vi "SVXMPL_Convert WDT to WAV.vi"(7 "Input range":sgl format="%.2f", 8 "error in (no error)":errorcluster, 10 "sound format":T1={"sound quality"=enum."mono", "rate"=enum."44100", "bits per sample"=enum."16 bit"}, 11 "Waveform":waveform(dbl)={"t0"=timestamp(0 s since 1904-01-01), "dt"=0.0, "Y"=[]}) -> (0 "error out":errorcluster, 2 "dup sound format":T1={"sound quality"=enum."mono", "rate"=enum."44100", "bits per sample"=enum."16 bit"}, 4 "gain":u16, 5 "mono 16-bit":i16[](array[numeric]), 6 "Coerced range":u16)   [LabVIEW 2017]
uses:
  <vilib>/sound/lvsound.llb/Sound Format.ctl
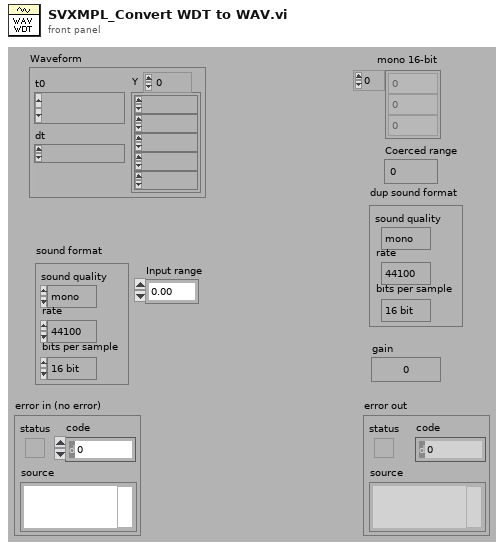
[diagram p1: front panel]
types:
  T1 = typedef "Sound Format.ctl" = cluster{"sound quality":enum16{"mono", "stereo"}, "rate":enum16{"11025", "22050", "44100", "8000"}, "bits per sample":enum16{"8 bit", "16 bit"}}
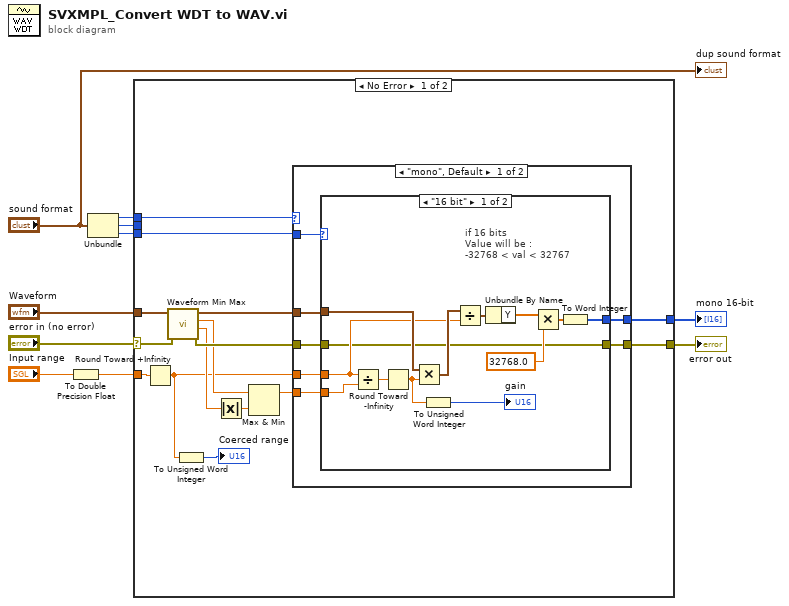
[diagram p0: block diagram]
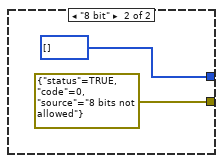
[diagram p2: hidden frame]
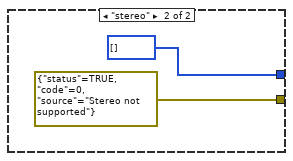
[diagram p3: hidden frame]
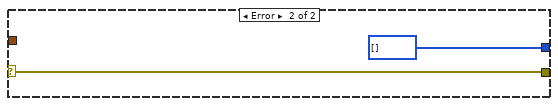
[diagram p4: hidden frame]
diagram:
  n1 = To Double Precision Float(number="Input range") -> (double precision float=w2:dbl)
  n2 = Unbundle("sound format") -> ("sound quality"=w7:enum16{"mono", "stereo"}, "rate"=w6:enum16{"11025", "22050", "44100", "8000"}, "bits per sample"=w9:enum16{"8 bit", "16 bit"})
  n3 = case shown="No Error" "error in (no error)" {
    selector: "error in (no error)" -> [w20 w50]
    tunnel: w7 -> [w25 _]
    tunnel: w9 -> [w24 _]
    tunnel: w6 -> [_ _]
    tunnel: "Waveform" -> [w22 _]
    tunnel: [w23 i16[] []] -> w4
    tunnel: w2 -> [w12 _]
    tunnel: [w14 w50] -> w1
    frame No Error {
      n4 = Round Toward +Infinity(x=w12) -> (ceil(x): smallest int >= x=w11:dbl)
      n5 = call <vilib>:"Waveform Min Max.vi"("error in (no error)"=w20, "waveform in"=w22) -> ("error out"=w19:errorcluster, "Y min"=w18:dbl, "Y max"=w17:dbl, "waveform out"=w21:waveform(dbl))  [unwired: 4 in, 2 out]
      n6 = To Unsigned Word Integer(number=w11) -> (unsigned 16bit integer=→"Coerced range":u16)
      n7 = Absolute Value(x=w18) -> (abs(x)=w16:dbl)
      n8 = Max & Min(x=w17, y=w16) -> (max(x,y)=w15:dbl)  [unwired: 1 out]
      n9 = case shown="\"mono\", Default" w25 {
        tunnel: w24 -> [w32 _]
        tunnel: [w30 i16[] []] -> w23
        tunnel: w21 -> [w31 _]
        tunnel: w11 -> [w29 _]
        tunnel: w19 -> [w27 _]
        tunnel: w15 -> [w28 _]
        tunnel: [w26 errorcluster {"status"=TRUE, "code"=0, "source"="Stereo not supported"} ("error out")] -> w14
        frame "mono", Default {
          n10 = case shown="\"16 bit\"" w32 {
            tunnel: [w42 i16[] []] -> w30
            tunnel: w31 -> [w39 _]
            tunnel: w29 -> [w37 _]
            tunnel: w28 -> [w36 _]
            tunnel: w27 -> [w35 _]
            tunnel: [w35 errorcluster {"status"=TRUE, "code"=0, "source"="8 bits not allowed"} ("error out")] -> w26
            frame "16 bit" {
              # "if 16 bits\nValue will be :\n-32768 < val < 32767"
              n11 = Divide(x=w37, y=w36) -> (x/y=w40:dbl)
              n12 = Round Toward -Infinity(1:w40) -> (0:w34:dbl)
              n13 = Multiply(x=w39, y=w34) -> (x*y=w38:waveform(dbl))
              n14 = To Unsigned Word Integer(number=w34) -> (unsigned 16bit integer=→"gain":u16)
              n15 = Divide(x=w38, y=w37) -> (x/y=w41:waveform(dbl))
              n16 = Unbundle By Name(w41) -> ("Y"=w43:dbl[])
              n17 = Multiply(x=w43, y=32768.0 ("ratio")) -> (x*y=w44:dbl[])
              n18 = To Word Integer(number=w44) -> (16bit integer=w42:i16[])
            }
            frame "8 bit" {
            }
          }
        }
        frame "stereo" {
        }
      }
    }
    frame Error {
    }
  }
  "error out" <- w1
  "mono 16-bit" <- w4
  "dup sound format" <- "sound format"
